vi "Main_FPGA_4.vi"() -> ()   [LabVIEW 2017]
uses:
  <vilib>/eio/EIONode/EIONode.xnode
  <vilib>/rvi/eio/common/nirviEmuTemplateMethod_errors.vi
  <vilib>/rvi/DataTransferAndStorage/Container/XNode/niFpgaContainer.xnode
  <vilib>/rvi/interface/RandomDataEmulation/nirviRandomDataFpgaMultiElementTemplate.vi
  <vilib>/eio/EIOPropertyNode/EIOPropertyNode.xnode
  <vilib>/rvi/eio/common/nirviEmuTemplatePropertyGet_errors.vi
  <vilib>/rvi/eio/common/nirviEmuTemplatePropertyGet_noerrors.vi
  <vilib>/rvi/eio/common/nirviEmuTemplatePropertySet_errors.vi
  <vilib>/rvi/eio/common/nirviEmuTemplatePropertySet_noerrors.vi
  <vilib>/eio/EIOMethodNode/EIOMethodNode.xnode
  <vilib>/LabVIEW Targets/FPGA/cRIO/shared/nicrio_ModuleControls/nicrio_cRIO-9770_DataRatesRing.ctl
panel:
  out "Chassis Temperature":sgl
  in  "Tab Control":enum32{"Dev 1", "Dev 2", "Dev 3", "Dev 4"}(tab)
  out "Data Over-Run 1":bool
  out "Error 1":errorcluster
  out "LO Frequency (Hz) 1":u32
  out "Downconverter Gain (dB) 1":fxp<+/-,15,8>
  out "PeakRFPower 1":fxp<+/-,12,8>
  in  "AcqSettings.Ch 1":T2={"Center Frequency (Hz)"=10000000, "Data Rate"=0, "Number of Samples"=1000, "Continuous"=FALSE, "Reference Level (dBm)"=0.0} {"Data Rate" items=["320.000 kS/s (NI 9770)", "256.000 kS/s (NI 9770)", "128.000 kS/s (NI 9770)", "64.000 kS/s (NI 9770)", "32.000 kS/s (NI 9770)", "16.000 kS/s (NI 9770)", "8.000 kS/s (NI 9770)", "4.000 kS/s (NI 9770)"]; "Center Frequency (Hz)" format="%.0p"}
  in  "Start 1":bool
  in  "Stop 1":bool
  in  "Start 2":bool
  in  "AcqSettings.Ch 2":T2={"Center Frequency (Hz)"=10000000, "Data Rate"=0, "Number of Samples"=1000, "Continuous"=FALSE, "Reference Level (dBm)"=0.0} {"Data Rate" items=["320.000 kS/s (NI 9770)", "256.000 kS/s (NI 9770)", "128.000 kS/s (NI 9770)", "64.000 kS/s (NI 9770)", "32.000 kS/s (NI 9770)", "16.000 kS/s (NI 9770)", "8.000 kS/s (NI 9770)", "4.000 kS/s (NI 9770)"]; "Center Frequency (Hz)" format="%.0p"}
  out "PeakRFPower 2":fxp<+/-,12,8>
  out "Data Over-Run 2":bool
  in  "Stop 2":bool
  out "Error 2":errorcluster
  out "LO Frequency (Hz) 2":u32
  out "Downconverter Gain (dB) 2":fxp<+/-,15,8>
  in  "Start 3":bool
  in  "AcqSettings.Ch 3":T2={"Center Frequency (Hz)"=10000000, "Data Rate"=0, "Number of Samples"=1000, "Continuous"=FALSE, "Reference Level (dBm)"=0.0} {"Data Rate" items=["320.000 kS/s (NI 9770)", "256.000 kS/s (NI 9770)", "128.000 kS/s (NI 9770)", "64.000 kS/s (NI 9770)", "32.000 kS/s (NI 9770)", "16.000 kS/s (NI 9770)", "8.000 kS/s (NI 9770)", "4.000 kS/s (NI 9770)"]; "Center Frequency (Hz)" format="%.0p"}
  out "PeakRFPower 3":fxp<+/-,12,8>
  out "Data Over-Run 3":bool
  in  "Stop 3":bool
  out "Error 3":errorcluster
  out "LO Frequency (Hz) 3":u32
  out "Downconverter Gain (dB) 3":fxp<+/-,15,8>
  in  "Start 4":bool
  in  "AcqSettings.Ch 4":T2={"Center Frequency (Hz)"=10000000, "Data Rate"=0, "Number of Samples"=1000, "Continuous"=FALSE, "Reference Level (dBm)"=0.0} {"Data Rate" items=["320.000 kS/s (NI 9770)", "256.000 kS/s (NI 9770)", "128.000 kS/s (NI 9770)", "64.000 kS/s (NI 9770)", "32.000 kS/s (NI 9770)", "16.000 kS/s (NI 9770)", "8.000 kS/s (NI 9770)", "4.000 kS/s (NI 9770)"]; "Center Frequency (Hz)" format="%.0p"}
  out "PeakRFPower 4":fxp<+/-,12,8>
  out "Data Over-Run 4":bool
  in  "Stop 4":bool
  out "Error 4":errorcluster
  out "LO Frequency (Hz) 4":u32
  out "Downconverter Gain (dB) 4":fxp<+/-,15,8>
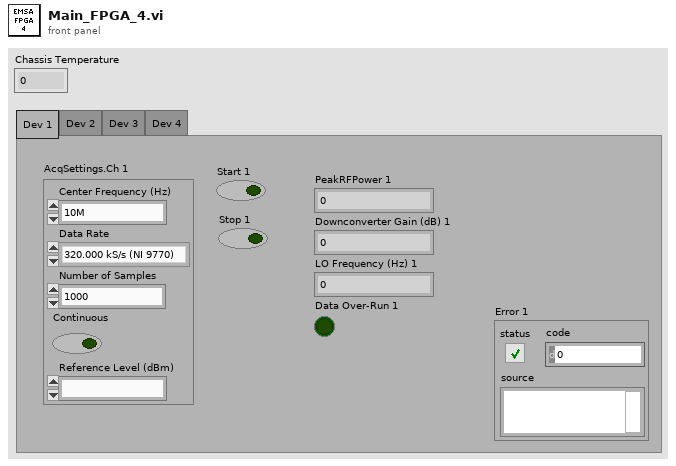
[diagram p1: front panel]
types:
  T1 = typedef "nicrio_cRIO-9770_DataRatesRing.ctl" = u8
  T2 = cluster{"Center Frequency (Hz)":u32, "Data Rate":T1, "Number of Samples":i32, "Continuous":bool, "Reference Level (dBm)":fxp<+/-,14,7>}
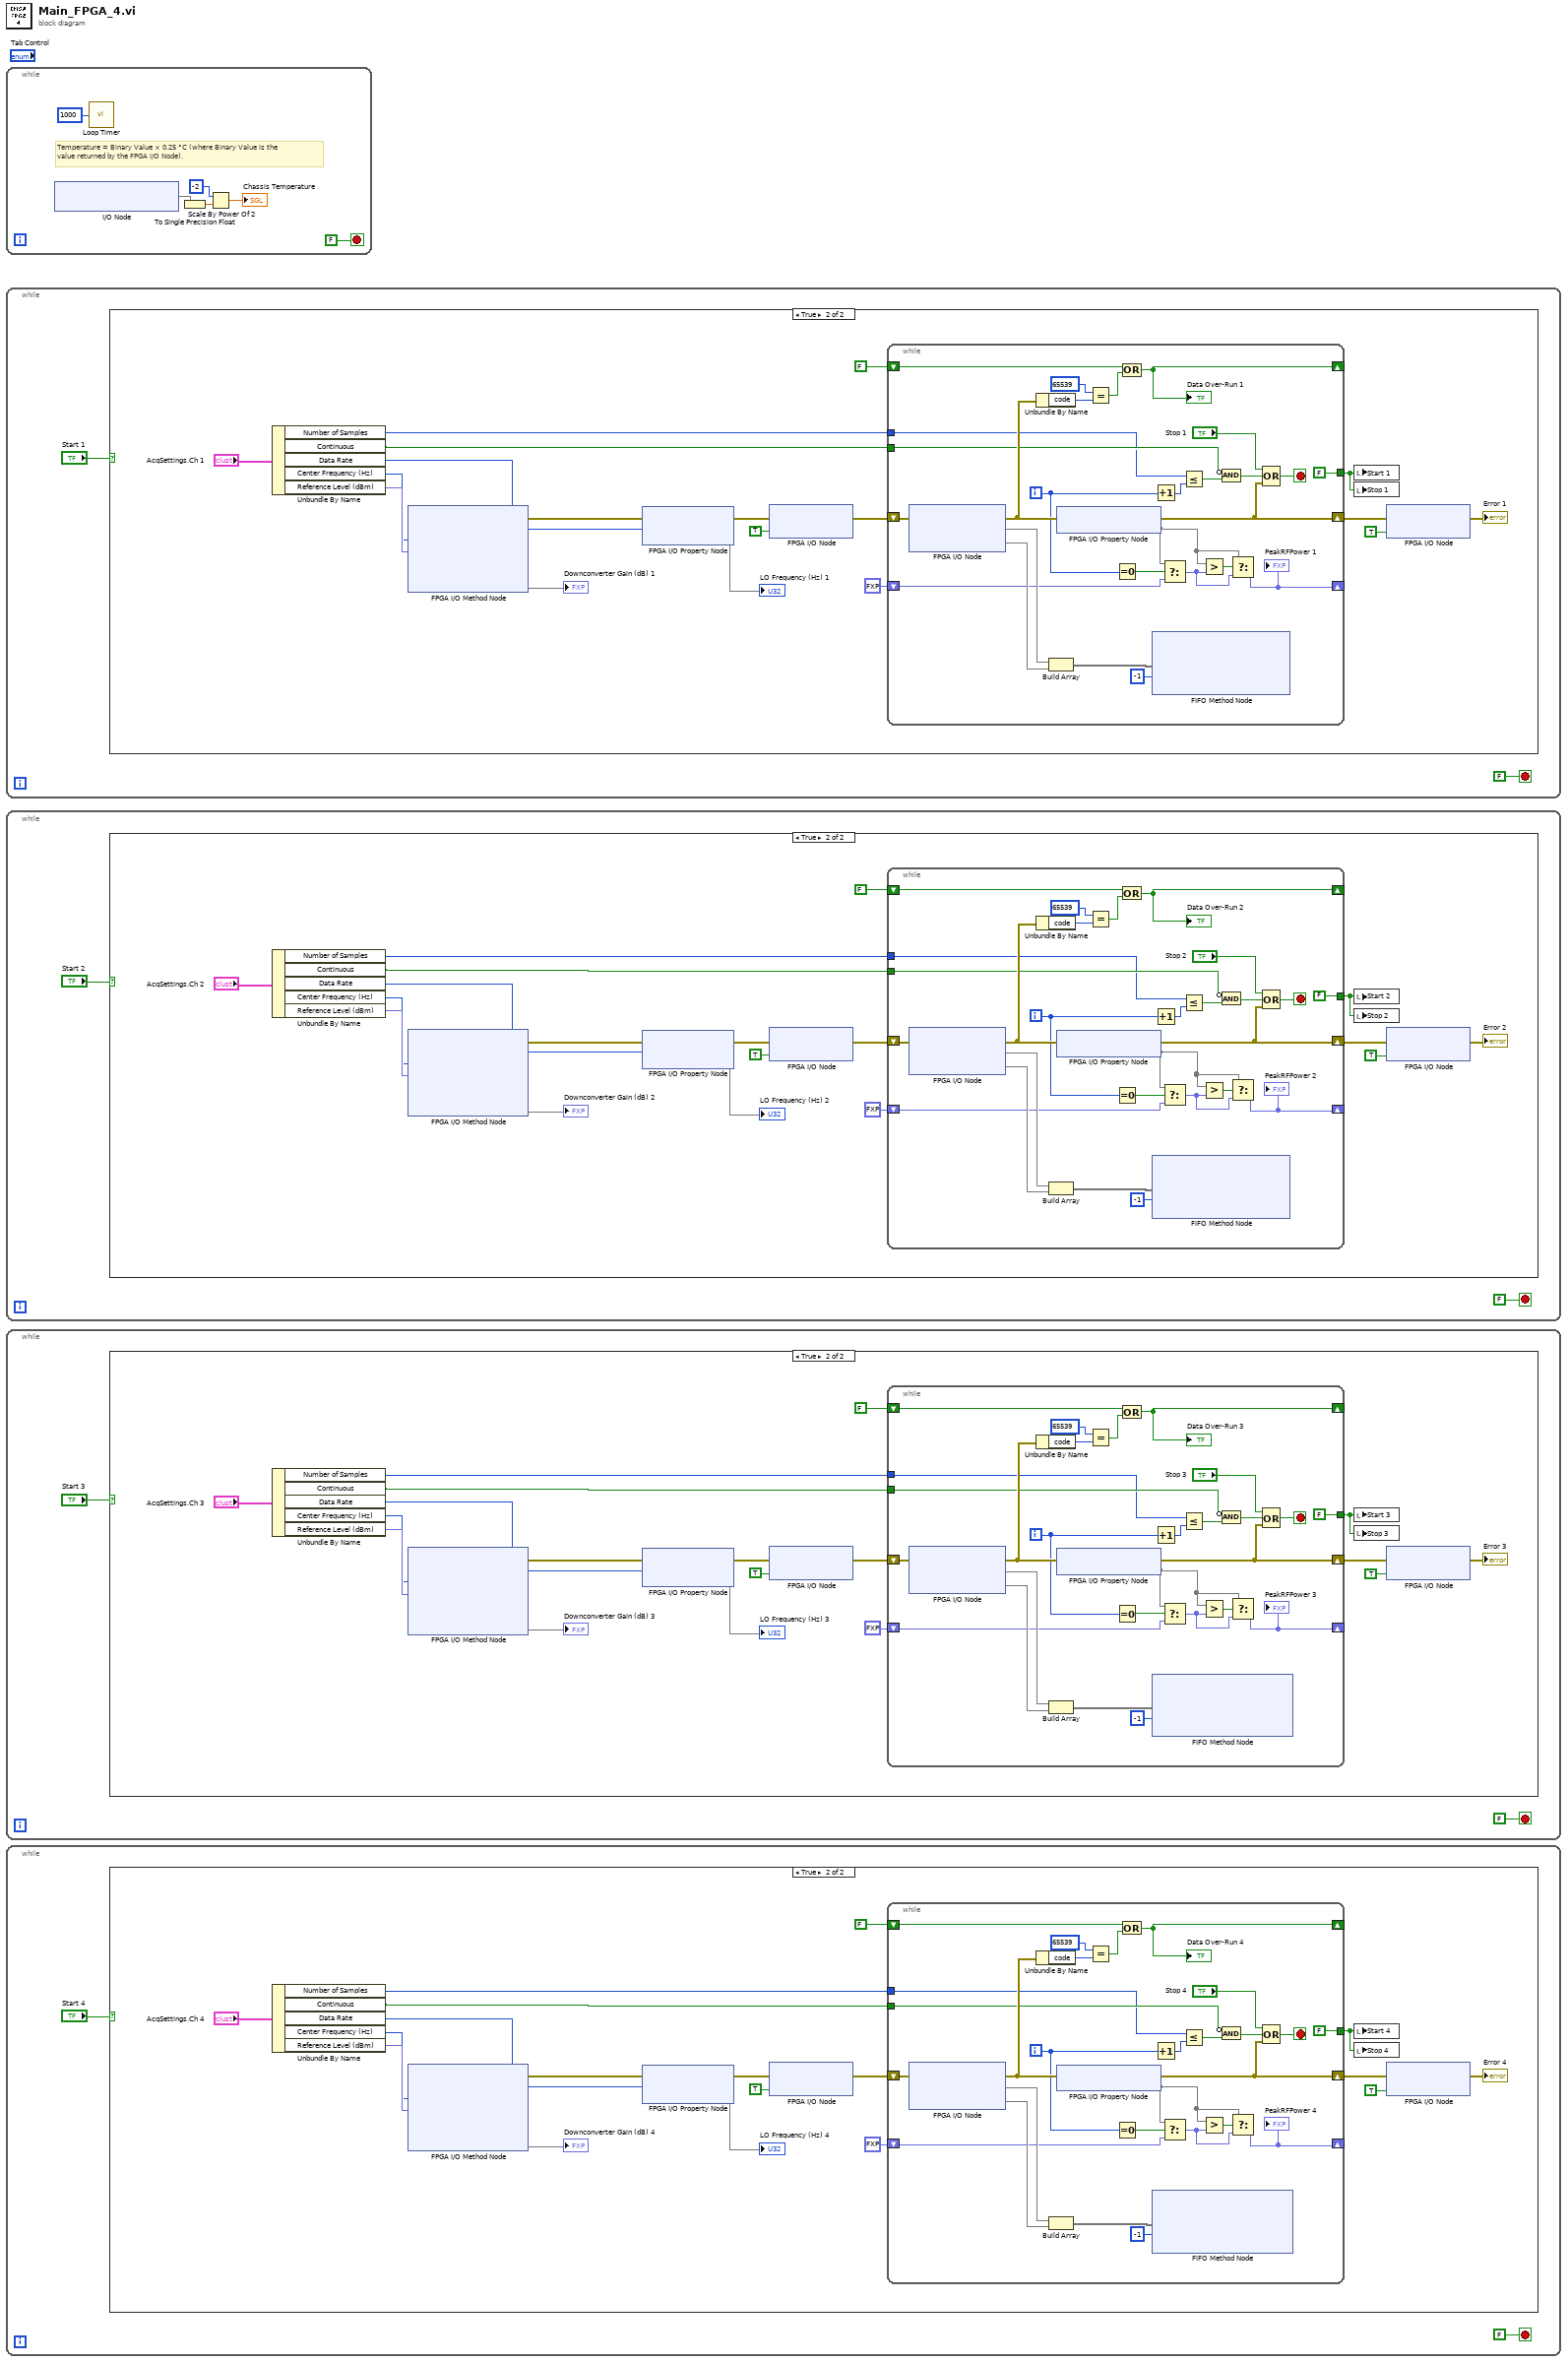
[diagram p0: block diagram]
diagram:
  n1 = while {
    stop <- FALSE stop-if-true
    # "Temperature = Binary Value × 0.25 °C (where Binary Value is the value returned by the FPGA I/O Node)."
    n2 = xnode "I/O Node"() -> ("Chassis Temperature"=w4)  [unwired: 1 in, 1 out]
    n3 = call "Loop Timer"("Count(mSec)"=u32 1000) -> ()  [unwired: 1 out]
    n4 = To Single Precision Float(number=w4) -> (single precision float=w6:sgl)
    n5 = Scale By Power Of 2(n=i16 -2, x=w6) -> (x*2^n=→"Chassis Temperature":sgl)
  }
  n6 = while {
    stop <- FALSE stop-if-true
    n7 = case shown="True" "Start 1" {
      frame False {
      }
      frame True {
        n8 = Unbundle By Name("AcqSettings.Ch 1") -> ("Number of Samples"=w10:i32, "Continuous"=w14:bool, "Data Rate"=w13:T1, "Center Frequency (Hz)"=w15:u32, "Reference Level (dBm)"=w16:fxp<+/-,14,7>)
        n9 = xnode "FPGA I/O Method Node"("Center Frequency"=w15, "Reference Level"=w16) -> ("error out"=w20:errorcluster, "Downconverter Gain"=→"Downconverter Gain (dB) 1")  [unwired: 4 in, 1 out]
        n10 = xnode "FPGA I/O Property Node"("error in"=w20, "Data Rate"=w13) -> ("error out"=w22:errorcluster, "LO Frequency"=→"LO Frequency (Hz) 1")  [unwired: 1 in, 1 out]
        n11 = xnode "FPGA I/O Node"("error in"=w22, "Mod1/Start"=TRUE ("start")) -> ("error out"=w21:errorcluster)  [unwired: 1 in, 1 out]
        n12 = while {
          shift-right: [w45] -> w25
          shift-left: w21 -> [w53]
          tunnel: [FALSE] -> w9
          shift-right: [w38] -> _
          shift-left: FALSE ("stop") -> [w40]
          shift-right: [w36] -> _
          shift-left: fxp<+/-,12,8> 0.0 ("Peak RF In Power") -> [w29]
          tunnel: w14 -> [w33]
          tunnel: w10 -> [w27]
          i -> [w31]
          stop <- w46 stop-if-true
          n13 = xnode "FPGA I/O Node"("error in"=w53) -> ("error out"=w43:errorcluster, "Mod1/RF In/I"=w52, "Mod1/RF In/Q"=w51)  [unwired: 2 in, 2 out]
          n14 = Unbundle By Name(w43) -> ("code"=w42:i32)
          n15 = Build Array(w52, w51) -> (w50:void[])
          n16 = xnode "FPGA I/O Property Node"("error in"=w43) -> ("error out"=w45:errorcluster, "Peak RF In Power"=w30)  [unwired: 1 in, 1 out]
          n17 = Equal?(x=65539, y=w42) -> (x = y?=w39:bool)
          n18 = Equal To 0?(x=w31) -> (x = 0?=w32:bool)
          n19 = Compound Arithmetic op=OR(w40, w39) -> (w38:bool)
          "Data Over-Run 1" <- w38
          n20 = xnode ("FIFO Method Node")("Element"=w50, "Timeout"=-1) -> ()  [unwired: 1 in, 2 out]
          n21 = Increment(x=w31) -> (x+1=w48:i32)
          n22 = Select(t=w30, s=w32, f=w29) -> (s? t:f=w28:fxp<+/-,12,8>)
          n23 = Less Or Equal?(x=w27, y=w48) -> (x <= y?=w35:bool)
          n24 = Greater?(x=w30, y=w28) -> (0:w37:bool)
          n25 = Compound Arithmetic op=AND(invert w33, w35) -> (w34:bool)
          n26 = Select(t=w30, s=w37, f=w28) -> (s? t:f=w36:fxp<+/-,12,8>)
          "PeakRFPower 1" <- w36
          n27 = Compound Arithmetic op=OR("Stop 1", w34, w45) -> (w46:bool)
        }
        n28 = local write "Start 1"(w9) -> ()
        n29 = local write "Stop 1"(w9) -> ()
        n30 = xnode "FPGA I/O Node"("error in"=w25, "Mod1/Stop"=TRUE ("stop")) -> ("error out"=→"Error 1":errorcluster)  [unwired: 1 in, 1 out]
      }
    }
  }
  n31 = while {
    stop <- FALSE stop-if-true
    n32 = case shown="True" "Start 2" {
      frame False {
      }
      frame True {
        n33 = Unbundle By Name("AcqSettings.Ch 2") -> ("Number of Samples"=w57:i32, "Continuous"=w61:bool, "Data Rate"=w60:T1, "Center Frequency (Hz)"=w62:u32, "Reference Level (dBm)"=w63:fxp<+/-,14,7>)
        n34 = xnode "FPGA I/O Method Node"("Center Frequency"=w62, "Reference Level"=w63) -> ("error out"=w67:errorcluster, "Downconverter Gain"=→"Downconverter Gain (dB) 2")  [unwired: 4 in, 1 out]
        n35 = xnode "FPGA I/O Property Node"("error in"=w67, "Data Rate"=w60) -> ("error out"=w69:errorcluster, "LO Frequency"=→"LO Frequency (Hz) 2")  [unwired: 1 in, 1 out]
        n36 = xnode "FPGA I/O Node"("error in"=w69, "Mod2/Start"=TRUE ("start")) -> ("error out"=w68:errorcluster)  [unwired: 1 in, 1 out]
        n37 = while {
          shift-right: [w92] -> w72
          shift-left: w68 -> [w100]
          tunnel: [FALSE] -> w56
          shift-right: [w85] -> _
          shift-left: FALSE ("stop") -> [w87]
          shift-right: [w83] -> _
          shift-left: fxp<+/-,12,8> 0.0 ("Peak RF In Power") -> [w76]
          tunnel: w61 -> [w80]
          tunnel: w57 -> [w74]
          i -> [w78]
          stop <- w93 stop-if-true
          n38 = xnode "FPGA I/O Node"("error in"=w100) -> ("error out"=w90:errorcluster, "Mod2/RF In/I"=w99, "Mod2/RF In/Q"=w98)  [unwired: 2 in, 2 out]
          n39 = Unbundle By Name(w90) -> ("code"=w89:i32)
          n40 = Build Array(w99, w98) -> (w97:void[])
          n41 = xnode "FPGA I/O Property Node"("error in"=w90) -> ("error out"=w92:errorcluster, "Peak RF In Power"=w77)  [unwired: 1 in, 1 out]
          n42 = Equal?(x=65539, y=w89) -> (x = y?=w86:bool)
          n43 = Equal To 0?(x=w78) -> (x = 0?=w79:bool)
          n44 = Compound Arithmetic op=OR(w87, w86) -> (w85:bool)
          "Data Over-Run 2" <- w85
          n45 = xnode ("FIFO Method Node")("Element"=w97, "Timeout"=-1) -> ()  [unwired: 1 in, 2 out]
          n46 = Increment(x=w78) -> (x+1=w95:i32)
          n47 = Select(t=w77, s=w79, f=w76) -> (s? t:f=w75:fxp<+/-,12,8>)
          n48 = Less Or Equal?(x=w74, y=w95) -> (x <= y?=w82:bool)
          n49 = Greater?(x=w77, y=w75) -> (0:w84:bool)
          n50 = Compound Arithmetic op=AND(invert w80, w82) -> (w81:bool)
          n51 = Select(t=w77, s=w84, f=w75) -> (s? t:f=w83:fxp<+/-,12,8>)
          "PeakRFPower 2" <- w83
          n52 = Compound Arithmetic op=OR("Stop 2", w81, w92) -> (w93:bool)
        }
        n53 = local write "Start 2"(w56) -> ()
        n54 = local write "Stop 2"(w56) -> ()
        n55 = xnode "FPGA I/O Node"("error in"=w72, "Mod2/Stop"=TRUE ("stop")) -> ("error out"=→"Error 2":errorcluster)  [unwired: 1 in, 1 out]
      }
    }
  }
  n56 = while {
    stop <- FALSE stop-if-true
    n57 = case shown="True" "Start 3" {
      frame False {
      }
      frame True {
        n58 = Unbundle By Name("AcqSettings.Ch 3") -> ("Number of Samples"=w104:i32, "Continuous"=w108:bool, "Data Rate"=w107:T1, "Center Frequency (Hz)"=w109:u32, "Reference Level (dBm)"=w110:fxp<+/-,14,7>)
        n59 = xnode "FPGA I/O Method Node"("Center Frequency"=w109, "Reference Level"=w110) -> ("error out"=w114:errorcluster, "Downconverter Gain"=→"Downconverter Gain (dB) 3")  [unwired: 4 in, 1 out]
        n60 = xnode "FPGA I/O Property Node"("error in"=w114, "Data Rate"=w107) -> ("error out"=w116:errorcluster, "LO Frequency"=→"LO Frequency (Hz) 3")  [unwired: 1 in, 1 out]
        n61 = xnode "FPGA I/O Node"("error in"=w116, "Mod3/Start"=TRUE ("start")) -> ("error out"=w115:errorcluster)  [unwired: 1 in, 1 out]
        n62 = while {
          shift-right: [w139] -> w119
          shift-left: w115 -> [w147]
          tunnel: [FALSE] -> w103
          shift-right: [w132] -> _
          shift-left: FALSE ("stop") -> [w134]
          shift-right: [w130] -> _
          shift-left: fxp<+/-,12,8> 0.0 ("Peak RF In Power") -> [w123]
          tunnel: w108 -> [w127]
          tunnel: w104 -> [w121]
          i -> [w125]
          stop <- w140 stop-if-true
          n63 = xnode "FPGA I/O Node"("error in"=w147) -> ("error out"=w137:errorcluster, "Mod3/RF In/I"=w146, "Mod3/RF In/Q"=w145)  [unwired: 2 in, 2 out]
          n64 = Unbundle By Name(w137) -> ("code"=w136:i32)
          n65 = Build Array(w146, w145) -> (w144:void[])
          n66 = xnode "FPGA I/O Property Node"("error in"=w137) -> ("error out"=w139:errorcluster, "Peak RF In Power"=w124)  [unwired: 1 in, 1 out]
          n67 = Equal?(x=65539, y=w136) -> (x = y?=w133:bool)
          n68 = Equal To 0?(x=w125) -> (x = 0?=w126:bool)
          n69 = Compound Arithmetic op=OR(w134, w133) -> (w132:bool)
          "Data Over-Run 3" <- w132
          n70 = xnode ("FIFO Method Node")("Element"=w144, "Timeout"=-1) -> ()  [unwired: 1 in, 2 out]
          n71 = Increment(x=w125) -> (x+1=w142:i32)
          n72 = Select(t=w124, s=w126, f=w123) -> (s? t:f=w122:fxp<+/-,12,8>)
          n73 = Less Or Equal?(x=w121, y=w142) -> (x <= y?=w129:bool)
          n74 = Greater?(x=w124, y=w122) -> (0:w131:bool)
          n75 = Compound Arithmetic op=AND(invert w127, w129) -> (w128:bool)
          n76 = Select(t=w124, s=w131, f=w122) -> (s? t:f=w130:fxp<+/-,12,8>)
          "PeakRFPower 3" <- w130
          n77 = Compound Arithmetic op=OR("Stop 3", w128, w139) -> (w140:bool)
        }
        n78 = local write "Start 3"(w103) -> ()
        n79 = local write "Stop 3"(w103) -> ()
        n80 = xnode "FPGA I/O Node"("error in"=w119, "Mod3/Stop"=TRUE ("stop")) -> ("error out"=→"Error 3":errorcluster)  [unwired: 1 in, 1 out]
      }
    }
  }
  n81 = while {
    stop <- FALSE stop-if-true
    n82 = case shown="True" "Start 4" {
      frame False {
      }
      frame True {
        n83 = Unbundle By Name("AcqSettings.Ch 4") -> ("Number of Samples"=w151:i32, "Continuous"=w155:bool, "Data Rate"=w154:T1, "Center Frequency (Hz)"=w156:u32, "Reference Level (dBm)"=w157:fxp<+/-,14,7>)
        n84 = xnode "FPGA I/O Method Node"("Center Frequency"=w156, "Reference Level"=w157) -> ("error out"=w161:errorcluster, "Downconverter Gain"=→"Downconverter Gain (dB) 4")  [unwired: 4 in, 1 out]
        n85 = xnode "FPGA I/O Property Node"("error in"=w161, "Data Rate"=w154) -> ("error out"=w163:errorcluster, "LO Frequency"=→"LO Frequency (Hz) 4")  [unwired: 1 in, 1 out]
        n86 = xnode "FPGA I/O Node"("error in"=w163, "Mod4/Start"=TRUE ("start")) -> ("error out"=w162:errorcluster)  [unwired: 1 in, 1 out]
        n87 = while {
          shift-right: [w186] -> w166
          shift-left: w162 -> [w194]
          tunnel: [FALSE] -> w150
          shift-right: [w179] -> _
          shift-left: FALSE ("stop") -> [w181]
          shift-right: [w177] -> _
          shift-left: fxp<+/-,12,8> 0.0 ("Peak RF In Power") -> [w170]
          tunnel: w155 -> [w174]
          tunnel: w151 -> [w168]
          i -> [w172]
          stop <- w187 stop-if-true
          n88 = xnode "FPGA I/O Node"("error in"=w194) -> ("error out"=w184:errorcluster, "Mod4/RF In/I"=w193, "Mod4/RF In/Q"=w192)  [unwired: 2 in, 2 out]
          n89 = Unbundle By Name(w184) -> ("code"=w183:i32)
          n90 = Build Array(w193, w192) -> (w191:void[])
          n91 = xnode "FPGA I/O Property Node"("error in"=w184) -> ("error out"=w186:errorcluster, "Peak RF In Power"=w171)  [unwired: 1 in, 1 out]
          n92 = Equal?(x=65539, y=w183) -> (x = y?=w180:bool)
          n93 = Equal To 0?(x=w172) -> (x = 0?=w173:bool)
          n94 = Compound Arithmetic op=OR(w181, w180) -> (w179:bool)
          "Data Over-Run 4" <- w179
          n95 = xnode ("FIFO Method Node")("Element"=w191, "Timeout"=-1) -> ()  [unwired: 1 in, 2 out]
          n96 = Increment(x=w172) -> (x+1=w189:i32)
          n97 = Select(t=w171, s=w173, f=w170) -> (s? t:f=w169:fxp<+/-,12,8>)
          n98 = Less Or Equal?(x=w168, y=w189) -> (x <= y?=w176:bool)
          n99 = Greater?(x=w171, y=w169) -> (0:w178:bool)
          n100 = Compound Arithmetic op=AND(invert w174, w176) -> (w175:bool)
          n101 = Select(t=w171, s=w178, f=w169) -> (s? t:f=w177:fxp<+/-,12,8>)
          "PeakRFPower 4" <- w177
          n102 = Compound Arithmetic op=OR("Stop 4", w175, w186) -> (w187:bool)
        }
        n103 = local write "Start 4"(w150) -> ()
        n104 = local write "Stop 4"(w150) -> ()
        n105 = xnode "FPGA I/O Node"("error in"=w166, "Mod4/Stop"=TRUE ("stop")) -> ("error out"=→"Error 4":errorcluster)  [unwired: 1 in, 1 out]
      }
    }
  }
